vi "STATESERIAL.vi"() -> ()   [LabVIEW 2014]
uses:
  STATE_DEMO.ctl
  libSerial/stateSerialUltra.ctl
panel:
  in  "IN COM":refnum<visa-resource-name>
  in  "error out":errorcluster
  out "X":dbl
  out "Z":dbl
  out "Y":dbl
  out "STATUS":enum16{"Running", "Waiting", "Pos", "IDLE"}(ring)
  out "DATA GET":string
  out "QUEUE GET":string
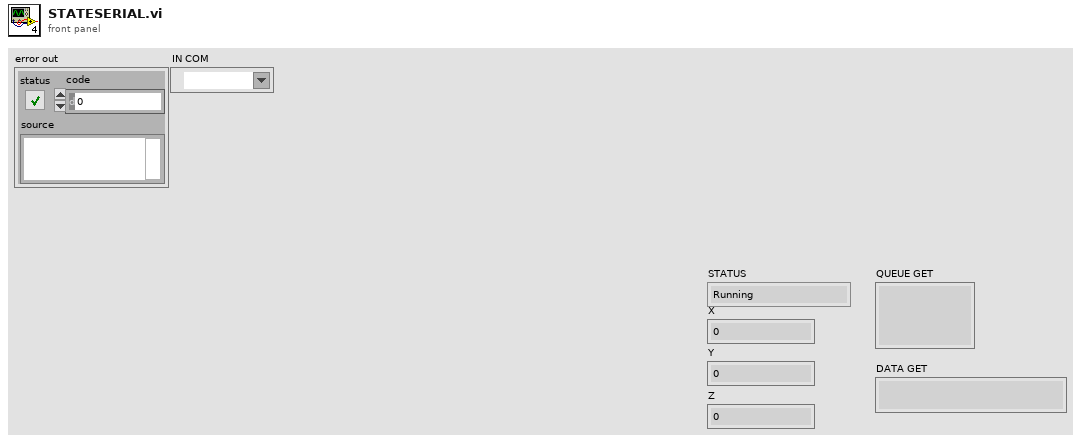
[diagram p1: front panel]
types:
  T1 = typedef "STATE_DEMO.ctl" = enum16{"INIT_STATE", "SEND_STATE", "GET_STATE", "STOP_STATE", "IDLE _STATE", "GET_QUEUE", "Decode_data"}
  T2 = typedef "stateSerialUltra.ctl" = enum16{"findCOM", "Init", "CheckConnect", "Read", "Write", "exit"}
  T3 = cluster{"Enum":enum16{"Running", "Waiting", "Pos", "IDLE"}, "X":dbl, "Y":dbl, "Z":dbl}
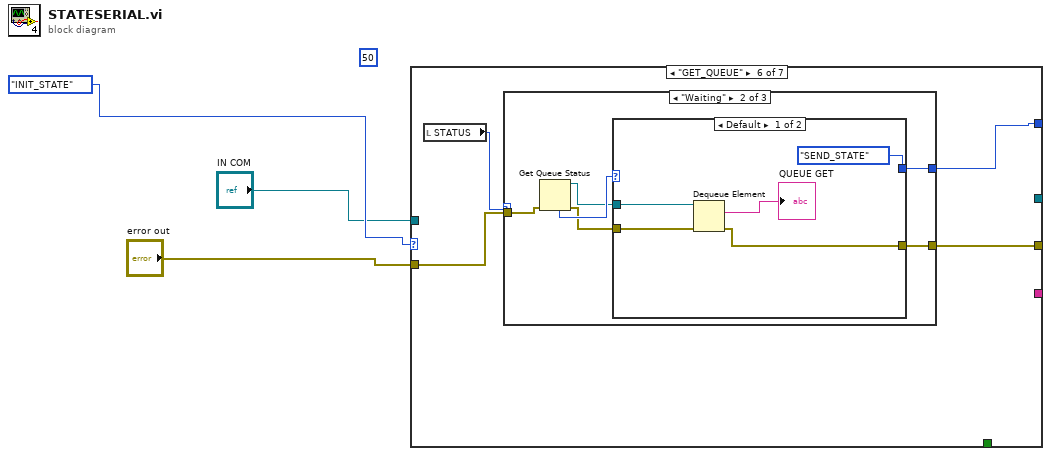
[diagram p0: block diagram]
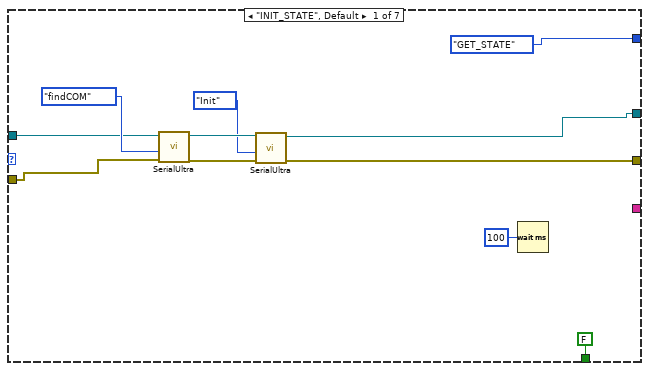
[diagram p2: hidden frame]
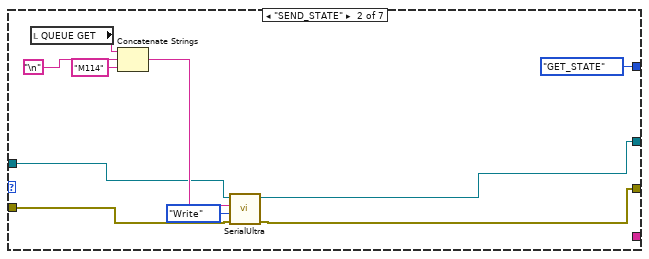
[diagram p3: hidden frame]
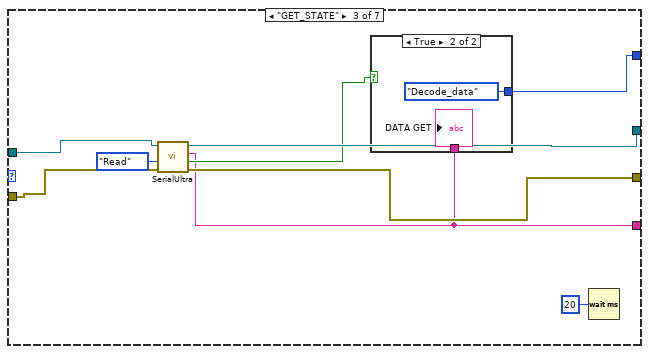
[diagram p4: hidden frame]
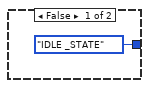
[diagram p5: hidden frame]
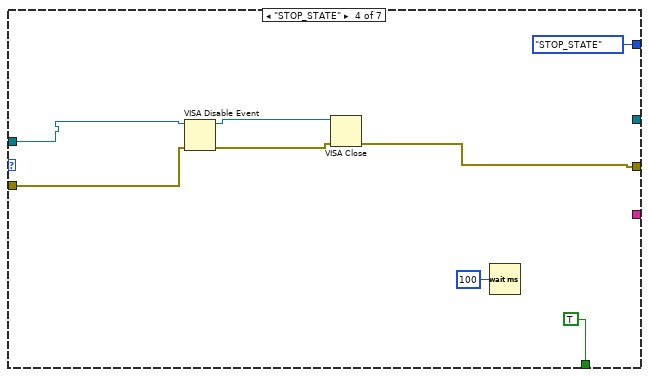
[diagram p6: hidden frame]
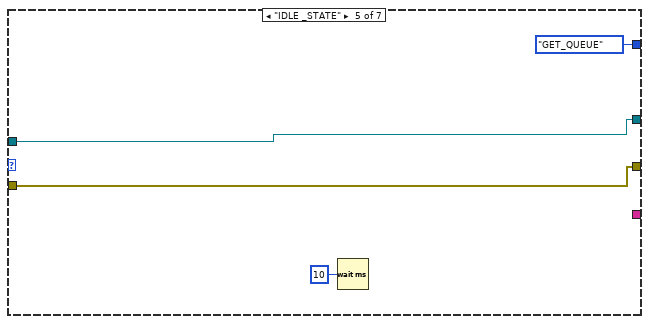
[diagram p7: hidden frame]
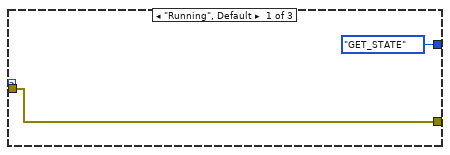
[diagram p8: hidden frame]
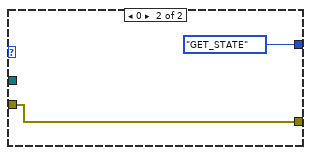
[diagram p9: hidden frame]
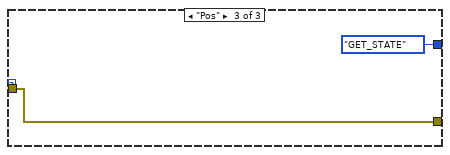
[diagram p10: hidden frame]
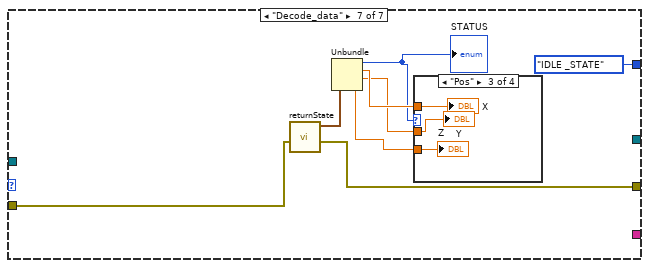
[diagram p11: hidden frame]
diagram:
  (unwired) 50
  n1 = case shown="\"GET_QUEUE\"" STATE_DEMO."INIT_STATE" ("STATE") {
    tunnel: [w7 w17 w30 _ w45 _ w78] -> _
    tunnel: [STATE_DEMO."GET_STATE" ("STATE") STATE_DEMO."GET_STATE" ("STATE") w27 STATE_DEMO."STOP_STATE" ("STATE") STATE_DEMO."GET_QUEUE" ("STATE") w51 STATE_DEMO."IDLE _STATE" ("STATE")] -> _
    tunnel: [w6 w16 w29 w41 w48 w50 w74] -> _
    tunnel: "error out" -> [w5 w20 w32 w44 w48 w52 w76]
    tunnel: [FALSE _ _ TRUE _ _ _] -> _
    tunnel: [_ _ w26 _ _ _ w77] -> _
    tunnel: "IN COM" -> [w4 w15 w25 w37 w45 _ _]
    frame "INIT_STATE", Default {
      n2 = call "SerialUltra.vi"("error in"=w5, "State"=stateSerialUltra."findCOM", "IN COM"=w4) -> ("error out"=w9:errorcluster, "OUT COM 2"=w10:refnum<visa-resource-name>)  [unwired: 4 in, 3 out]
      n3 = call "SerialUltra.vi"("error in"=w9, "State"=stateSerialUltra."Init", "IN COM"=w10) -> ("error out"=w6:errorcluster, "OUT COM 2"=w7:refnum<visa-resource-name>)  [unwired: 4 in, 3 out]
      n4 = Wait (ms)(milliseconds to wait=u32 100) -> ()  [unwired: 1 out]
    }
    frame "SEND_STATE" {
      n5 = local read "QUEUE GET"() -> (w23:string)
      n6 = Concatenate Strings(w23, "\n", "M114" ("string")) -> (w19:string)
      n7 = call "SerialUltra.vi"("error in"=w20, "State"=stateSerialUltra."Write", "Data Write"=w19, "IN COM"=w15) -> ("error out"=w16:errorcluster, "OUT COM 2"=w17:refnum<visa-resource-name>)  [unwired: 3 in, 3 out]
    }
    frame "GET_STATE" {
      n8 = call "SerialUltra.vi"("error in"=w32, "State"=stateSerialUltra."Read", "IN COM"=w25) -> ("error out"=w29:errorcluster, "IsData"=w28:bool, "DataOut"=w26:string, "OUT COM 2"=w30:refnum<visa-resource-name>)  [unwired: 4 in, 1 out]
      n9 = case shown="True" w28 {
        tunnel: [STATE_DEMO."IDLE _STATE" ("STATE") STATE_DEMO."Decode_data" ("STATE")] -> w27
        tunnel: w26 -> [_ w35]
        frame False {
        }
        frame True {
          "DATA GET" <- w35
        }
      }
      n10 = Wait (ms)(milliseconds to wait=u32 20) -> ()  [unwired: 1 out]
    }
    frame "STOP_STATE" {
      n11 = VISA Disable Event(8:w44, 11:w37) -> (0:w42:errorcluster, 3:w43:refnum<visa-resource-name>)  [unwired: 2 in]
      n12 = VISA Close(VISA resource name=w43, error in (no error)=w42) -> (error out=w41:errorcluster)
      n13 = Wait (ms)(milliseconds to wait=u32 100) -> ()  [unwired: 1 out]
    }
    frame "IDLE _STATE" {
      n14 = Wait (ms)(milliseconds to wait=u32 10) -> ()  [unwired: 1 out]
    }
    frame "GET_QUEUE" {
      n15 = local read "STATUS"() -> (w49:enum16{"Running", "Waiting", "Pos", "IDLE"})
      n16 = case shown="\"Waiting\"" w49 {
        tunnel: w52 -> [w54 w60 w69]
        tunnel: [STATE_DEMO."GET_STATE" ("STATE") w58 STATE_DEMO."GET_STATE" ("STATE")] -> w51
        tunnel: [w54 w55 w69] -> w50
        frame "Running", Default {
        }
        frame "Waiting" {
          n17 = Get Queue Status(error in (no error)=w60) -> (queue out=w57:refnum<queue>, error out=w56:errorcluster, # elements in queue=w59:i32)  [unwired: 2 in, 5 out]
          n18 = case shown="Default" w59 {
            tunnel: [STATE_DEMO."SEND_STATE" ("STATE") STATE_DEMO."GET_STATE" ("STATE")] -> w58
            tunnel: w57 -> [w65 _]
            tunnel: w56 -> [w64 w66]
            tunnel: [w63 w66] -> w55
            frame Default {
              n19 = Dequeue Element(queue=w65, error in (no error)=w64) -> (element=→"QUEUE GET":string, error out=w63:errorcluster)  [unwired: 1 in, 2 out]
            }
            frame 0 {
            }
          }
        }
        frame "Pos" {
        }
      }
    }
    frame "Decode_data" {
      n20 = call "returnState.vi"("error IN"=w76) -> ("error out"=w74:errorcluster, "output cluster"=w75:T3)  [unwired: 9 in]
      n21 = Unbundle(w75) -> ("Enum"=w70:enum16{"Running", "Waiting", "Pos", "IDLE"}, "X"=w73:dbl, "Y"=w72:dbl, "Z"=w71:dbl)
      "STATUS" <- w70
      n22 = case shown="\"Pos\"" w70 {
        tunnel: w73 -> [_ _ w82 _]
        tunnel: w72 -> [_ _ w81 _]
        tunnel: w71 -> [_ _ w80 _]
        frame "Running", Default {
        }
        frame "Waiting" {
        }
        frame "Pos" {
          "Y" <- w81
          "Z" <- w80
          "X" <- w82
        }
        frame "IDLE" {
        }
      }
    }
  }
